vi "Read LoopStopCondition.vi"(8 "error in (no error)":errorcluster, 11 "Test in":refnum<class "Test.lvclass">) -> (0 "error out":errorcluster, 2 "LoopStopCondition":T1, 3 "Test out":refnum<class "Test.lvclass">)   [LabVIEW 2014, in "Test.lvclass"]
uses:
  Test.lvclass
  Typedef/LoopStopCondition.ctl
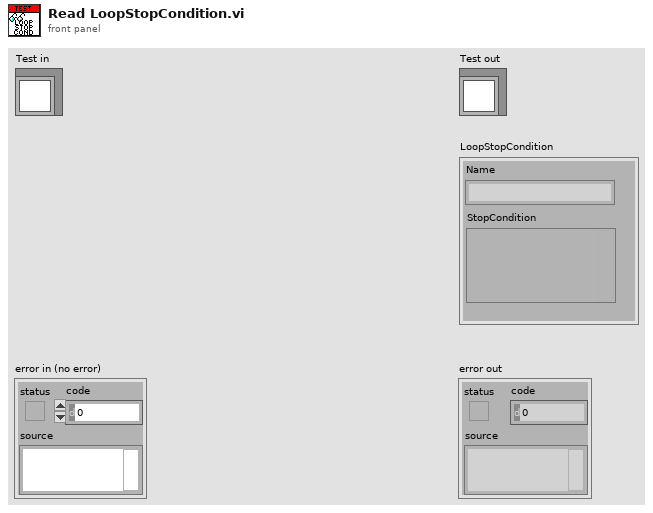
[diagram p1: front panel]
types:
  T1 = typedef "Test.lvclass/LoopStopCondition.ctl" = cluster{"Name":string, "StopCondition":variant}
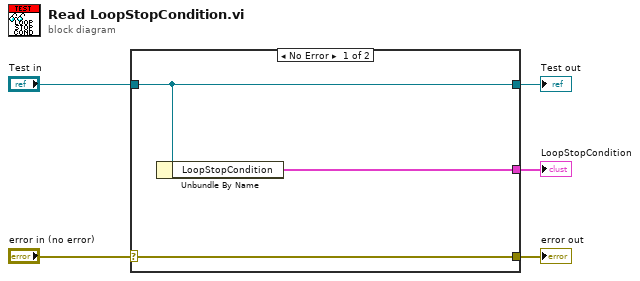
[diagram p0: block diagram]
diagram:
  n1 = case shown="No Error" "error in (no error)" {
    selector: "error in (no error)" -> [w8 w9]
    tunnel: [w8 w9] -> w4
    tunnel: [w7 w10] -> w2
    tunnel: "Test in" -> [w7 w10]
    tunnel: [w6 _] -> w1
    frame No Error {
      n2 = Unbundle By Name(w7) -> ("LoopStopCondition"=w6:T1)
    }
    frame Error {
    }
  }
  "error out" <- w4
  "Test out" <- w2
  "LoopStopCondition" <- w1
